vi "GetDigitalReference.vi"(8 "error in":errorcluster, 11 "Numeric Text in":refnum<class "Digital.lvclass">) -> (0 "error out":errorcluster, 1 "Digital reference":refnum<vi>, 3 "Numeric Text out":refnum<class "Digital.lvclass">)   [LabVIEW 2014, in "Digital.lvclass"]
uses:
  Digital.lvclass
  Generic/Generic.lvclass
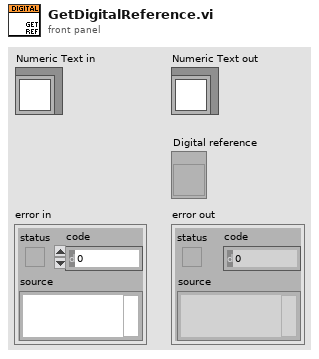
[diagram p1: front panel]
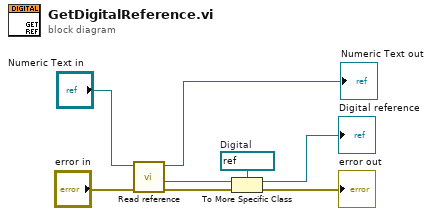
[diagram p0: block diagram]
diagram:
  w8 = refnum<vi> refnum  # Digital
  n1 = call "Read reference.vi"("error in"="error in", "GObject in"="Numeric Text in") -> ("error out"=w3:errorcluster, "reference"=w2:refnum<vi>, "GObject out"=→"Numeric Text out":refnum<class "Digital.lvclass">)  [unwired: 5 in]
  n2 = To More Specific Class(target class=w8, reference=w2, error in=w3) -> (specific class reference=→"Digital reference":refnum<vi>, error out=→"error out":errorcluster)
